vi "define columns.vi"(10 "Enum Array":refnum<vi>[](array[refnum])) -> (2 "Column Definition":T1[](array[typedef]) {"MinWidth" min=2 step=1; "AutoSizeMode" items=["None"=1, "ColumnHeader"=2, "AllCellsExceptHeader"=4, "AllCells"=6, "DisplayedCellsExceptHeader"=8, "DisplayedCells"=10, "Fill"=16]; "FillWeight" min=1 max=100})   [LabVIEW 2015, in "tag select module editor node.lvclass"]
uses:
  tag select module editor node.lvclass
  <vilib>/NI/DCAF/Tag Editor Core/Table API/Column/Column Descriptor.ctl
  <vilib>/NI/DCAF/Tag Editor Core/Table API/Column/Column.lvclass
  <vilib>/NI/DCAF/Tag Editor Core/Table API/Column/Column Type.ctl
  <vilib>/NI/Tag Bus/tag/Data Type.ctl
  <vilib>/NI/DCAF/Tag Editor Core/Table API/Table Manager/Call Back Ref Type Def.ctl
  <vilib>/NI/DCAF/Tag Editor Core/Configuration Editor/Classes/Engine Parent/Engine Parent Editor Node.lvclass
  <vilib>/NI/DCAF/Tag Editor Core/Configuration Editor/Classes/Module editor node/module editor node.lvclass
  Change Tag Select DT.vi
  Change Tag Output.vi
  Change Tag Select.vi
  Change Tag Input A.vi
  Change Tag Input B.vi
  <vilib>/NI/Tag Bus/tag/tag descriptor.lvclass
  <vilib>/NI/DCAF/Tag Editor Core/Table API/Mapping Column/Mapping Column.lvclass
  <vilib>/NI/DCAF/Tag Editor Core/Table API/String Column/String Column.lvclass
  <vilib>/NI/DCAF/Tag Editor Core/Table API/Listbox Enum Column/List Box Enum Column.lvclass
  <vilib>/NI/DCAF/Tag Editor Core/Table API/Table Manager/Table Manager.lvclass
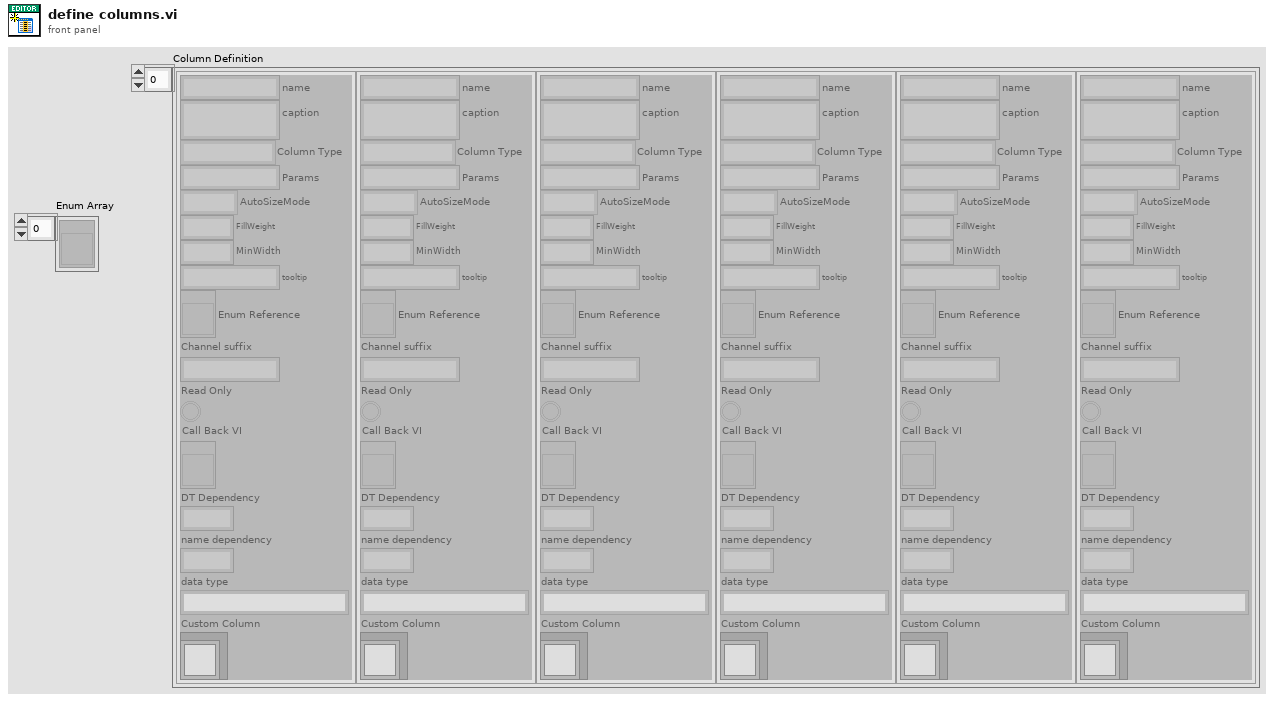
[diagram p1: front panel]
types:
  T1 = typedef "Table Manager.lvlib/Column.lvclass/Column Descriptor.ctl" = cluster{"name":string, "caption":string, "Column Type":T2, "Params":string, "AutoSizeMode":i32, "FillWeight":sgl, "MinWidth":u32, "tooltip":string, "Enum Reference":refnum<vi>, "Channel suffix":string, "Read Only":bool, "Call Back VI":T3, "DT Dependency":i32, "name dependency":i32, "data type":T4, "Custom Column":refnum<class "Column.lvclass">}
  T2 = typedef "Table Manager.lvlib/Column.lvclass/Column Type.ctl" = enum16{"String", "Mapping", "Enum", "Custom"}
  T3 = typedef "Table Manager.lvlib/Table Manager.lvclass/Call Back Ref Type Def.ctl" = refnum<vi>
  T4 = typedef "tag bus.lvlib/tag descriptor.lvclass/Data Type.ctl" = enum16{"Double", "Single", "I64", "I32", "I16", "I8", "U64", "U32", "U16", "U8", "Boolean", "String", "Array of Double", "Array of Single", "Array of I64", "Array of I32", "Array of I16", "Array of I8", "Array of U64", "Array of U32", "Array of U16", "Array of U8", "Array of Boolean", "Array of String"}
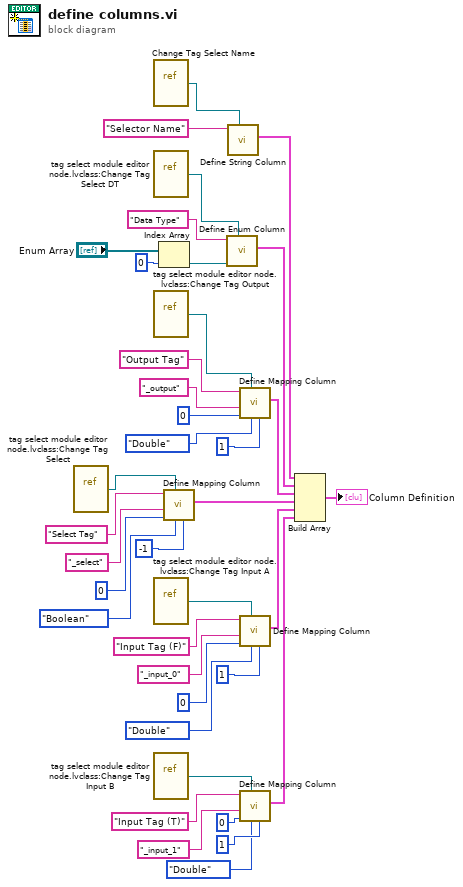
[diagram p0: block diagram]
diagram:
  n1 = vi-ref "tag select module editor node.lvclass:Change Tag Select.vi"() -> (w34:refnum<vi>)
  n2 = vi-ref "Change Tag Select Name.vi"() -> (w3:refnum<vi>)
  n3 = vi-ref "tag select module editor node.lvclass:Change Tag Select DT.vi"() -> (w6:refnum<vi>)
  n4 = vi-ref "tag select module editor node.lvclass:Change Tag Output.vi"() -> (w33:refnum<vi>)
  n5 = vi-ref "tag select module editor node.lvclass:Change Tag Input A.vi"() -> (w35:refnum<vi>)
  n6 = vi-ref "tag select module editor node.lvclass:Change Tag Input B.vi"() -> (w36:refnum<vi>)
  n7 = Index Array(array="Enum Array", index=0) -> (element=w7:refnum<vi>)
  n8 = call <vilib>:"Define Mapping Column.vi"("DT Dependency (-1)"=-1 ("DT Dependency"), "data type"=Data_Type."Boolean", "Call Back VI"=w34, "name dependency"=0, "Channel suffix"="_select" ("string"), "name"="Select Tag") -> ("Column Descriptor out"=w22:T1)  [unwired: 5 in]
  n9 = call <vilib>:"Define Enum Column.vi"("Call Back VI"=w6, "Enum Reference"=w7, "Name"="Data Type" ("name")) -> ("Column Descriptor out"=w5:T1)  [unwired: 8 in]
  n10 = call <vilib>:"Define String Column.vi"("Call Back VI"=w3, "Name"="Selector Name" ("name")) -> ("Column Descriptor out"=w2:T1)  [unwired: 9 in]
  n11 = call <vilib>:"Define Mapping Column.vi"("DT Dependency (-1)"=1 ("DT Dependency"), "data type"=Data_Type."Double", "Call Back VI"=w33, "name dependency"=0, "Channel suffix"="_output" ("string"), "name"="Output Tag") -> ("Column Descriptor out"=w32:T1)  [unwired: 5 in]
  n12 = call <vilib>:"Define Mapping Column.vi"("DT Dependency (-1)"=1 ("DT Dependency"), "data type"=Data_Type."Double", "Call Back VI"=w35, "name dependency"=0, "Channel suffix"="_input_0" ("string"), "name"="Input Tag (F)") -> ("Column Descriptor out"=w12:T1)  [unwired: 5 in]
  n13 = call <vilib>:"Define Mapping Column.vi"("DT Dependency (-1)"=1 ("DT Dependency"), "data type"=Data_Type."Double", "Call Back VI"=w36, "name dependency"=0, "Channel suffix"="_input_1" ("string"), "name"="Input Tag (T)") -> ("Column Descriptor out"=w23:T1)  [unwired: 5 in]
  n14 = Build Array(w2, w5, w32, w22, w12, w23) -> (→"Column Definition":T1[])
